vi "FA_DateString_to_TimeStamp.vi"(11 "DateTime String":string) -> (3 "Time Stamp":timestamp=timestamp(3403656258 s since 1904-01-01))   [LabVIEW 2014, in "FA_FIRST.lvlib"]
uses:
  FA_FIRST.lvlib
  <vilib>/Utility/miscctls.llb/LVDateTimeRec.ctl
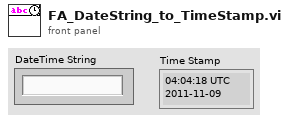
[diagram p1: front panel]
types:
  T1 = typedef "LVDateTimeRec.ctl" = cluster{"fractional second":dbl, "second":i32, "minute":i32, "hour":i32, "day of month":i32, "month":i32, "year":i32, "day of week":i32, "day of year":i32, "DST":i32}
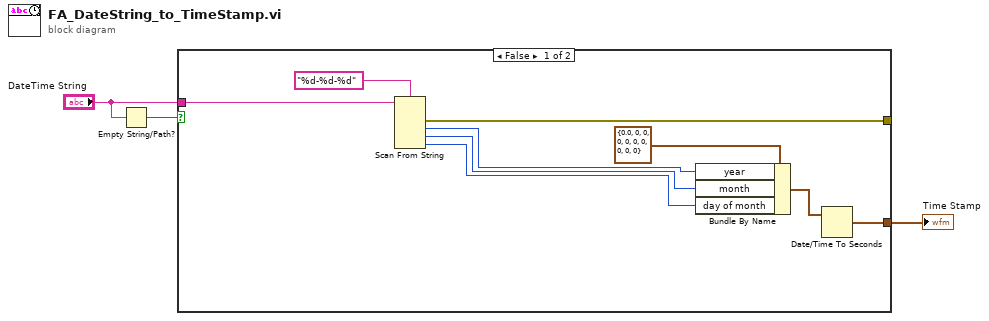
[diagram p0: block diagram]
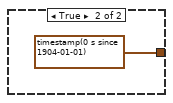
[diagram p2: hidden frame]
diagram:
  n1 = Empty String/Path?(string/path="DateTime String") -> (empty?=w3:bool)
  n2 = case shown="False" w3 {
    tunnel: [w4 timestamp(0 s since 1904-01-01)] -> w2
    tunnel: "DateTime String" -> [w12 _]
    tunnel: [w10 _] -> _
    frame False {
      n3 = Scan From String(format string="%d-%d-%d", input string=w12) -> (error out=w10:errorcluster, output 1=w8:i32, output 2=w7:i32, output 3=w6:i32)  [unwired: 5 in, 2 out]
      n4 = Bundle By Name(cluster=T1 {"fractional second"=0.0, "second"=0, "minute"=0, "hour"=0, "day of month"=0, "month"=0, "year"=0, "day of week"=0, "day of year"=0, "DST"=0} ("date time rec"), "year"=w8, "month"=w7, "day of month"=w6) -> (w5:T1)
      n5 = Date/Time To Seconds(2:w5) -> (0:w4:timestamp)  [unwired: 1 in]
    }
    frame True {
    }
  }
  "Time Stamp" <- w2
